vi "Begin.vi"() -> (0 "error out":errorcluster)   [LabVIEW 2013]
doc: "Called before other user functions, this VI is expected to open initial I/O refnums, load in file data, and do all program initialization. Notice that the <B>error out</B> terminal is simply used for data flow. Wiring it to other structures or subVIs ensures that this VI runs first."
uses:
  <vilib>/Rock Robotics/WPI/SafetyOutput/WPI_SafetyOutputConfigMenu.ctl
  <vilib>/Rock Robotics/WPI/DriverStation/WPI_DriverStationRobotMode2.ctl
  <vilib>/Rock Robotics/WPI/Joystick/WPI_JoystickDeviceEnum.ctl
  <vilib>/Rock Robotics/SystemInterfaces/DIO/FPGA_DIOPWMChannel.ctl
  <vilib>/Rock Robotics/SystemInterfaces/DIO/FPGA_DIOChannel.ctl
  Robot Global Data.vi
  <vilib>/Rock Robotics/WPI/RobotDrive/WPI_RobotDriveOpen4MotorWithJaguar.vi
  <vilib>/Rock Robotics/WPI/MotorControl/WPI_MotorControlOpen Jaguar.vi
  <vilib>/Rock Robotics/WPI/Joystick/WPI_JoystickDevRef.ctl
panel:
  out "error out 2":errorcluster
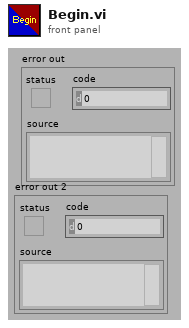
[diagram p1: front panel]
types:
  T1 = typedef "FPGA_DIOPWMChannel.ctl" = enum8{"PWM 1", "PWM 2", "PWM 3", "PWM 4", "PWM 5", "PWM 6", "PWM 7", "PWM 8", "PWM 9", "PWM 10", "Invalid"}
  T2 = typedef "FPGA_DIOChannel.ctl" = enum8{"DIO 1", "DIO 2", "DIO 3", "DIO 4", "DIO 5", "DIO 6", "DIO 7", "DIO 8", "DIO 9", "DIO 10", "DIO 11", "DIO 12", "DIO 13", "DIO 14", "Invalid"}
  T3 = typedef "WPI_JoystickDeviceEnum.ctl" = enum16{"USB 1", "USB 2", "USB 3", "USB 4", "Kinect 1", "Kinect 2"}
  T4 = typedef "WPI_DriverStationRobotMode2.ctl" = enum16{"Autonomous Disabled", "Autonomous Enabled", "Teleop Disabled", "Teleop Enabled", "Timeout", "Finish", "Test Disabled", "Test Enabled"}
  T5 = typedef "WPI_SafetyOutputConfigMenu.ctl" = enum16{"Enable", "Disable"}
  T6 = typedef "WPI_JoystickDevRef.ctl" = cluster{"Device":T3}
  T7 = typedef "WPI_JoystickButtonState.ctl" = cluster{"Button 1":bool, "Button 2":bool, "Button 3":bool, "Button 4":bool, "Button 5":bool, "Button 6":bool, "Button 7":bool, "Button 8":bool, "Button 9":bool, "Button 10":bool, "Button 11":bool, "Button 12":bool}
  T8 = cluster{"axis 1 (x)":dbl, "axis 2 (y)":dbl, "axis 3 (throttle)":dbl, "axis 4":dbl, "axis 5":dbl, "axis 6":dbl}
  T9 = typedef "WPI_DigitalInputDevRef.ctl" = cluster{"DevStatus":errorcluster, "DIO Channel":T2, "Digital Module":T10}
  T10 = typedef "FPGA_TypedefDigitalModule.ctl" = enum16{"Digital Module 1", "Digital Module 2"}
  T11 = typedef "WPI_ServoDeviceRef.ctl" = cluster{"DeviceStatus":errorcluster, "Digital Module":T10, "PWM Channel":T1, "DeadBand":T12}
  T12 = typedef "WPI_PWMDeadband.ctl" = cluster{"Name":string, "maxPositivePwm":i32, "minPositivePwm":i32, "centerPwm":i32, "maxNegativePwm":i32, "minNegativePwm":i32, "angularRange":u16}
  T13 = typedef "WPI_MotorControlDeviceRef.ctl" = cluster{"DeviceStatus":errorcluster, "Type":enum16{"PWM", "CAN"}, "PWM":cluster{"Digital Module":T10, "PWM Channel":T1, "DeadBand":T12}, "CAN":cluster{"Device Number":u8, "Control Mode":T14, "Semaphore":T15, "Max Vout":dbl}, "Invert":bool, "TransformRef":T16, "InvTransformRef":T16}
  T14 = typedef "WPI_CANJaguar_ControlMode.ctl" = enum8{"Percent VBus", "Current", "Speed", "Position", "Voltage"}
  T15 = typedef "Semaphore RefNum" = refnum<k1>
  T16 = typedef "WPI_PWMTransform_ConPane.ctl" = refnum<vi>
  T17 = typedef "WPI_RobotDriveDevRef.ctl" = cluster{"DevStatus":errorcluster, "Motors[]":T13[], "Square Inputs":bool, "Max Output":dbl, "Isochronous":bool}
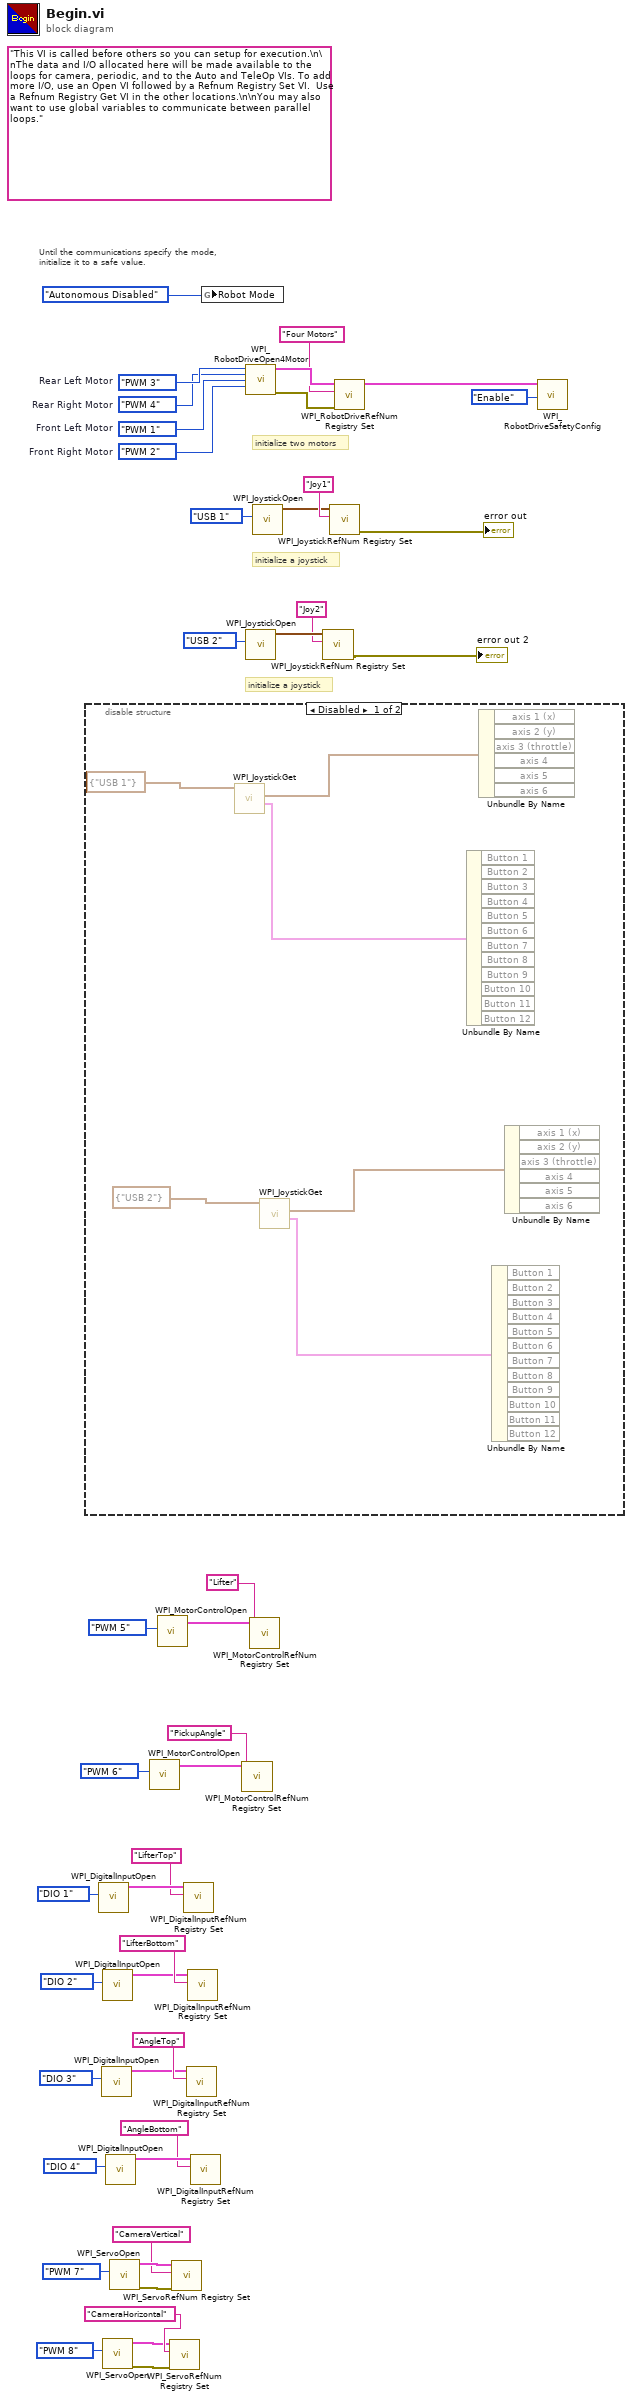
[diagram p0: block diagram]
diagram:
  w32 = FPGA_DIOPWMChannel."PWM 2"  # Front Right Motor
  w33 = FPGA_DIOPWMChannel."PWM 1"  # Front Left Motor
  w34 = FPGA_DIOPWMChannel."PWM 4"  # Rear Right Motor
  w35 = FPGA_DIOPWMChannel."PWM 3"  # Rear Left Motor
  (unwired) "This VI is called before others so you can setup for execution.\n\nThe data and I/O allocated here will be made available to the loops for camera, periodic, and to the Auto and TeleOp VIs. To add more I/O, use an Open VI followed by a Refnum Registry Set VI.  Use a Refnum Registry Get VI in the other locations.\n\nYou may also want to use global variables to communicate between parallel loops."
  # "initialize a joystick"
  # "initialize a joystick"
  # "Until the communications specify the mode,\ninitialize it to a safe value."
  # "initialize two motors"
  n1 = disable-structure shown="Disabled" {
    frame Disabled {
      n2 = call <vilib>:"WPI_JoystickGet.vi"("JoystickDevRef"=T6 {"Device"=enum."USB 1"}) -> ("Buttons"=w48:T7, "Axes"=w49:T8)  [unwired: 4 in, 1 out]
      n3 = call <vilib>:"WPI_JoystickGet.vi"("JoystickDevRef"=T6 {"Device"=enum."USB 2"}) -> ("Buttons"=w47:T7, "Axes"=w46:T8)  [unwired: 4 in, 1 out]
      n4 = Unbundle By Name(w48) -> ()  [unwired: 12 out]
      n5 = Unbundle By Name(w49) -> ()  [unwired: 6 out]
      n6 = Unbundle By Name(w47) -> ()  [unwired: 12 out]
      n7 = Unbundle By Name(w46) -> ()  [unwired: 6 out]
    }
    frame Enabled {
    }
  }
  n8 = call <vilib>:"WPI_DigitalInputOpen.vi"("DIO Channel"=FPGA_DIOChannel."DIO 1") -> ("DigitalInputDevRef"=w19:T9)  [unwired: 9 in, 1 out]
  n9 = call <vilib>:"WPI_DigitalInputOpen.vi"("DIO Channel"=FPGA_DIOChannel."DIO 3") -> ("DigitalInputDevRef"=w10:T9)  [unwired: 9 in, 1 out]
  n10 = call <vilib>:"WPI_DigitalInputOpen.vi"("DIO Channel"=FPGA_DIOChannel."DIO 2") -> ("DigitalInputDevRef"=w16:T9)  [unwired: 9 in, 1 out]
  n11 = call <vilib>:"WPI_ServoOpen.vi"("PWM Channel"=FPGA_DIOPWMChannel."PWM 8") -> ("error out"=w1:errorcluster, "ServoDeviceRef"=w2:T11)  [unwired: 9 in]
  n12 = call <vilib>:"WPI_DigitalInputOpen.vi"("DIO Channel"=FPGA_DIOChannel."DIO 4") -> ("DigitalInputDevRef"=w13:T9)  [unwired: 9 in, 1 out]
  n13 = call <vilib>:"WPI_ServoOpen.vi"("PWM Channel"=FPGA_DIOPWMChannel."PWM 7") -> ("error out"=w8:errorcluster, "ServoDeviceRef"=w7:T11)  [unwired: 9 in]
  n14 = call-poly <vilib>:"WPI_MotorControlOpen.vi"("PWM Channel"=FPGA_DIOPWMChannel."PWM 6") -> ("MotorControlDeviceRef"=w22:T13)  [unwired: 9 in, 1 out]
  n15 = call-poly <vilib>:"WPI_MotorControlOpen.vi"("PWM Channel"=FPGA_DIOPWMChannel."PWM 5") -> ("MotorControlDeviceRef"=w25:T13)  [unwired: 9 in, 1 out]
  n16 = call <vilib>:"WPI_ServoRefNum Registry Set.vi"("error in (no error)"=w1, "refnum name"="CameraHorizontal", "ServoDeviceRef"=w2) -> ()  [unwired: 7 in, 2 out]
  n17 = call <vilib>:"WPI_ServoRefNum Registry Set.vi"("error in (no error)"=w8, "refnum name"="CameraVertical", "ServoDeviceRef"=w7) -> ()  [unwired: 7 in, 2 out]
  n18 = call <vilib>:"WPI_DigitalInputRefNum Registry Set.vi"("refnum name"="LifterTop", "DigitalInputDevRef"=w19) -> ()  [unwired: 8 in, 2 out]
  n19 = call <vilib>:"WPI_DigitalInputRefNum Registry Set.vi"("refnum name"="AngleTop", "DigitalInputDevRef"=w10) -> ()  [unwired: 8 in, 2 out]
  n20 = call <vilib>:"WPI_DigitalInputRefNum Registry Set.vi"("refnum name"="LifterBottom", "DigitalInputDevRef"=w16) -> ()  [unwired: 8 in, 2 out]
  n21 = call <vilib>:"WPI_DigitalInputRefNum Registry Set.vi"("refnum name"="AngleBottom", "DigitalInputDevRef"=w13) -> ()  [unwired: 8 in, 2 out]
  n22 = global write "Robot Global Data.vi" "Robot Mode"(WPI_DriverStationRobotMode2."Autonomous Disabled" ("Robot Mode")) -> ()
  n23 = call <vilib>:"WPI_MotorControlRefNum Registry Set.vi"("refnum name"="PickupAngle", "MotorControlDevRef"=w22) -> ()  [unwired: 8 in, 2 out]
  n24 = call-poly <vilib>:"WPI_RobotDriveOpen4Motor.vi"("Rear Left Motor"=w35, "Rear Right Motor"=w34, "Front Left Motor"=w33, "Front Right Motor"=w32) -> ("RobotDriveDevRef"=w44:T17, "error out"=w42:errorcluster)  [unwired: 10 in]
  n25 = call <vilib>:"WPI_JoystickOpen.vi"("JoystickDevice"=WPI_JoystickDeviceEnum."USB 2") -> ("JoystickDevRef"=w28:T6)  [unwired: 10 in]
  n26 = call <vilib>:"WPI_MotorControlRefNum Registry Set.vi"("refnum name"="Lifter", "MotorControlDevRef"=w25) -> ()  [unwired: 8 in, 2 out]
  n27 = call <vilib>:"WPI_JoystickOpen.vi"("JoystickDevice"=WPI_JoystickDeviceEnum."USB 1") -> ("JoystickDevRef"=w37:T6)  [unwired: 10 in]
  n28 = call <vilib>:"WPI_JoystickRefNum Registry Set.vi"("refnum name"="Joy2", "JoystickDevRef"=w28) -> ("error out"=→"error out 2":errorcluster)  [unwired: 8 in, 1 out]
  n29 = call <vilib>:"WPI_JoystickRefNum Registry Set.vi"("refnum name"="Joy1", "JoystickDevRef"=w37) -> ("error out"=→"error out":errorcluster)  [unwired: 8 in, 1 out]
  n30 = call <vilib>:"WPI_RobotDriveRefNum Registry Set.vi"("error in (no error)"=w42, "refnum name"="Four Motors", "RobotDriveDevRef"=w44) -> ("RobotDriveDevRef"=w41:T17)  [unwired: 8 out]
  n31 = call <vilib>:"WPI_RobotDriveSafetyConfig.vi"("mode"=WPI_SafetyOutputConfigMenu."Enable", "RobotDriveDevRef"=w41) -> ()  [unwired: 8 in, 2 out]
